vi "Populate all DIOs and AIOs in Enum.vi"(8 "error in (no error)":errorcluster) -> (0 "error out":errorcluster)   [LabVIEW 2013]
doc: "Copyright © 2005, Soliton Technologies.\nAll rights reserved."
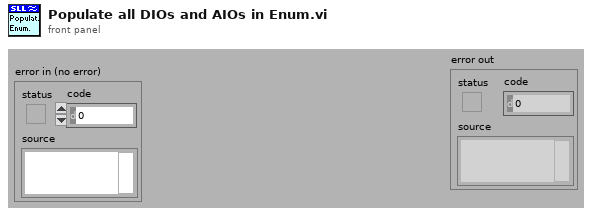
[diagram p1: front panel]
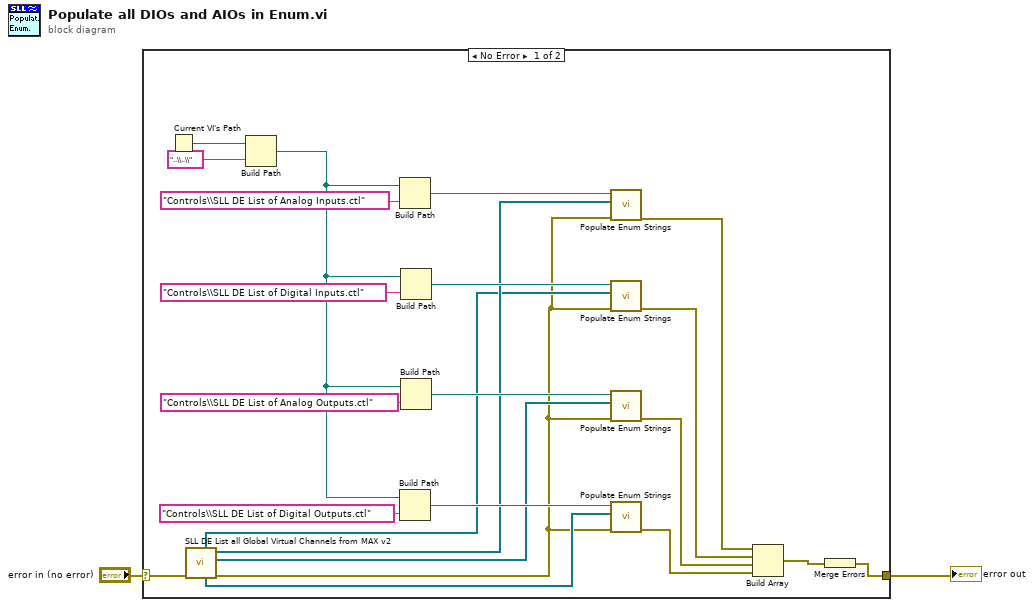
[diagram p0: block diagram]
diagram:
  n1 = case shown="No Error" "error in (no error)" {
    selector: "error in (no error)" -> [w16 w26]
    tunnel: [w18 w26] -> w1
    frame No Error {
      n2 = Current VI's Path() -> (path=w25:path)
      n3 = call "SLL DE List all Global Virtual Channels from MAX v2.vi"("error in (no error)"=w16) -> ("error out"=w3:errorcluster, "Analog Output"=w9:refnum<k21>[], "Analog Input"=w10:refnum<k21>[], "Digital Output"=w7:refnum<k21>[], "Digital Input"=w8:refnum<k21>[])  [unwired: 4 in, 2 out]
      n4 = Build Path(base path=w25, name or relative path="..\\..\\") -> (appended path=w11:path)
      n5 = Build Path(base path=w11, name or relative path="Controls\\SLL DE List of Analog Inputs.ctl") -> (appended path=w23:path)
      n6 = Build Path(base path=w11, name or relative path="Controls\\SLL DE List of Digital Outputs.ctl") -> (appended path=w20:path)
      n7 = Build Path(base path=w11, name or relative path="Controls\\SLL DE List of Digital Inputs.ctl") -> (appended path=w22:path)
      n8 = Build Path(base path=w11, name or relative path="Controls\\SLL DE List of Analog Outputs.ctl") -> (appended path=w21:path)
      n9 = call "Populate Enum Strings.vi"("error in (no error)"=w3, "Strings []"=w10, "Control Path"=w23) -> ("error out"=w4:errorcluster)  [unwired: 8 in]
      n10 = call "Populate Enum Strings.vi"("error in (no error)"=w3, "Strings []"=w8, "Control Path"=w22) -> ("error out"=w5:errorcluster)  [unwired: 8 in]
      n11 = call "Populate Enum Strings.vi"("error in (no error)"=w3, "Strings []"=w9, "Control Path"=w21) -> ("error out"=w6:errorcluster)  [unwired: 8 in]
      n12 = call "Populate Enum Strings.vi"("error in (no error)"=w3, "Strings []"=w7, "Control Path"=w20) -> ("error out"=w17:errorcluster)  [unwired: 8 in]
      n13 = Build Array(w4, w5, w6, w17) -> (w19:errorcluster[])
      n14 = Merge Errors(w19) -> (w18:errorcluster)
    }
    frame Error {
    }
  }
  "error out" <- w1
